vi "CheckM9.vi"(10 "Index":i32, 11 "Comm list":string[](array[string])) -> (3 "Gonna Stop Next":bool)   [LabVIEW 2016]
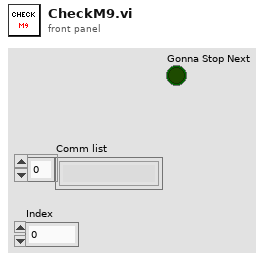
[diagram p1: front panel]
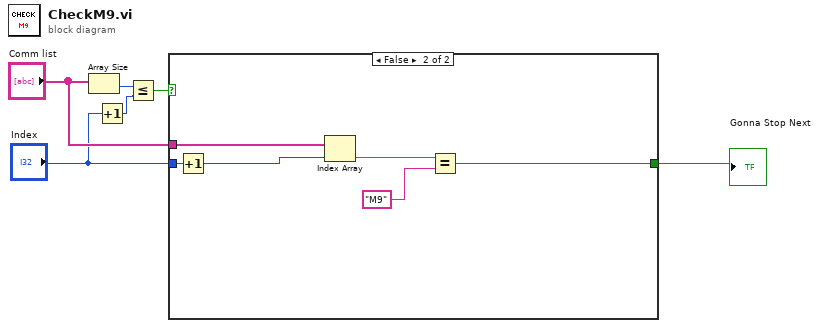
[diagram p0: block diagram]
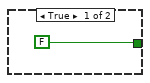
[diagram p2: hidden frame]
diagram:
  n1 = Array Size(array="Comm list") -> (size(s)=w5:i32)
  n2 = Increment(x="Index") -> (x+1=w2:i32)
  n3 = Less Or Equal?(x=w5, y=w2) -> (x <= y?=w4:bool)
  n4 = case shown="False" w4 {
    tunnel: "Index" -> [_ w13]
    tunnel: "Comm list" -> [_ w11]
    tunnel: [FALSE w8] -> w1
    frame True {
    }
    frame False {
      n5 = Increment(x=w13) -> (x+1=w12:i32)
      n6 = Index Array(array=w11, index=w12) -> (element=w10:string)
      n7 = Equal?(x=w10, y="M9") -> (x = y?=w8:bool)
    }
  }
  "Gonna Stop Next" <- w1
